vi "Common_Socket_Cmd_Sub_VI_TestMode.vi"(6 "Common Socket Error in":errorcluster, 8 "Operation Message Length":i32, 9 "Operation Message ID":i32, 11 "connection ID":refnum<k5>) -> (1 "error output":errorcluster, 3 "connection ID":refnum<k5>)   [LabVIEW 2017]
panel:
  out "Rest of the binary string":string
  out "bytes written":i32
  # "INPUT :"
  # "OUTPUT :"
  # "For Info :"
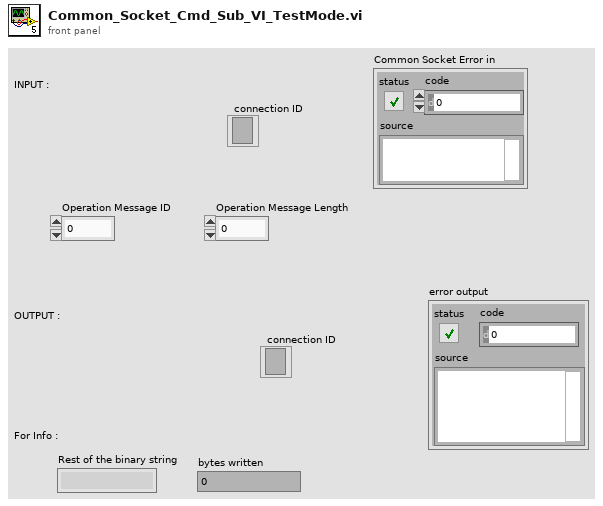
[diagram p1: front panel]
types:
  T1 = enum16{"big-endian, network order", "native, host order", "little-endian"}
  T2 = cluster{"Operation Message Length":i32, "Operation Message ID":i32}
  T3 = enum16{"Standard", "Buffered", "CRLF", "Immediate"}
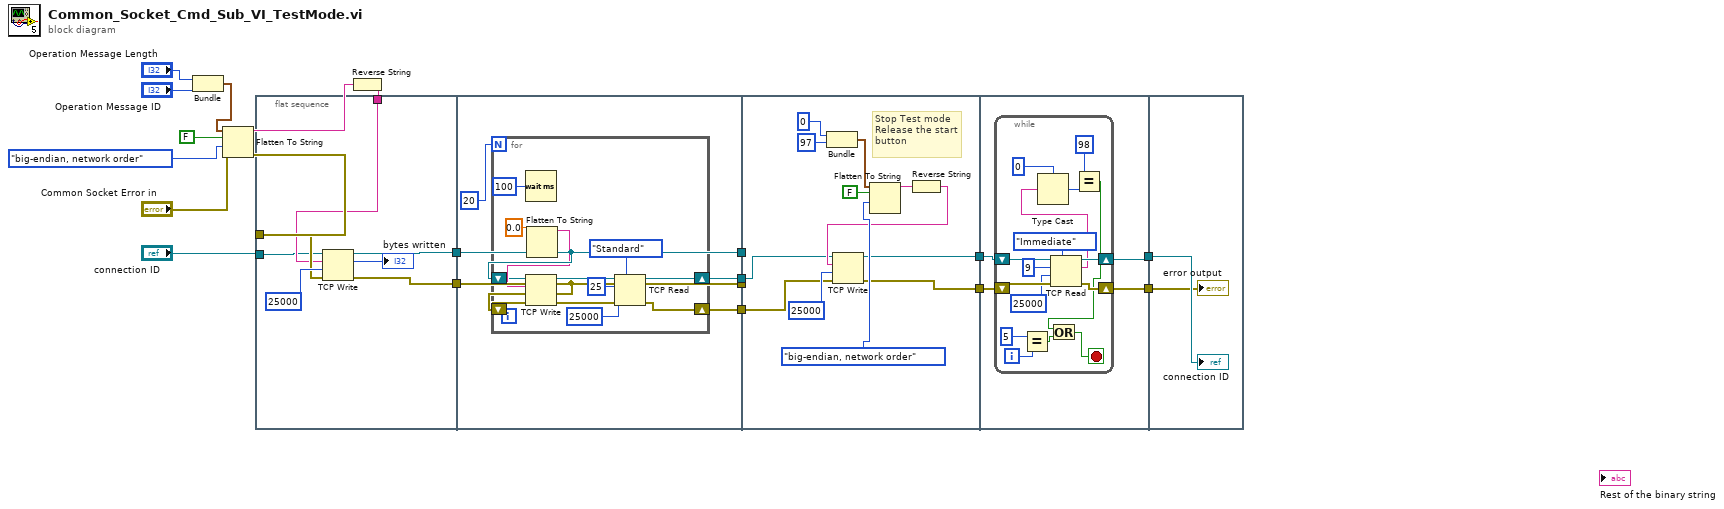
[diagram p0: block diagram]
diagram:
  n1 = Bundle("Operation Message Length"="Operation Message Length", "Operation Message ID"="Operation Message ID") -> (w13:T2)  [unwired: 1 in]
  n2 = Flatten To String(anything=w13, prepend array or string size? (T)=FALSE, byte order (0:big-endian, network order)=T1."big-endian, network order", error in (no error)="Common Socket Error in") -> (data string=w16:string, error out=w17:errorcluster)  [unwired: 1 out]
  n3 = flat-sequence {
    tunnel: [w25] -> w10
    tunnel: [w24] -> w8
    tunnel: w17 -> [w23]
    tunnel: w15 -> [w22]
    tunnel: "connection ID" -> [w21]
    tunnel: w10 -> [w32]
    tunnel: [w32] -> w9
    tunnel: w8 -> [w31]
    tunnel: [w31] -> w7
    tunnel: [w29] -> w6
    tunnel: [w28] -> w5
    tunnel: w9 -> [_]
    tunnel: w7 -> [_]
    tunnel: [w48] -> w4
    tunnel: [w47] -> w2
    tunnel: w6 -> [w46]
    tunnel: w5 -> [w45]
    tunnel: w4 -> [w60]
    tunnel: [w58] -> w3
    tunnel: w2 -> [w59]
    tunnel: [w57] -> w1
    tunnel: w3 -> [w78]
    tunnel: w1 -> [w77]
    frame #0 {
      n4 = TCP Write(connection ID=w21, data in=w22, error in (no error)=w23, 9:25000 ("timeout ms (25000)")) -> (connection ID out=w25:refnum<k5>, bytes written=→"bytes written":i32, error out=w24:errorcluster)
    }
    frame #1 {
      n5 = for {
        N: 20 -> [_]
        shift-right: [w38] -> w29
        shift-left: w32 -> [w43]
        shift-right: [w36] -> w28
        shift-left: w31 -> [w42]
        n6 = Wait (ms)(milliseconds to wait=u32 100) -> ()  [unwired: 1 out]
        n7 = Flatten To String(anything=0.0) -> (data string=w44:string)  [unwired: 3 in, 2 out]
        n8 = TCP Write(connection ID=w43, data in=w44, error in (no error)=w42) -> (connection ID out=w39:refnum<k5>, error out=w37:errorcluster)  [unwired: 1 in, 1 out]
        n9 = TCP Read(connection ID=w39, bytes to read=25, error in (no error)=w37, 7:T3."Standard" ("mode (standard)"), 9:25000 ("timeout ms (25000)")) -> (connection ID out=w38:refnum<k5>, error out=w36:errorcluster)  [unwired: 1 out]
      }
    }
    frame #2 {
      # "Stop Test mode\nRelease the start\nbutton"
      n10 = Bundle(0, 97) -> (w55:cluster{i32, i32})  [unwired: 1 in]
      n11 = Flatten To String(anything=w55, prepend array or string size? (T)=FALSE, byte order (0:big-endian, network order)=T1."big-endian, network order") -> (data string=w56:string)  [unwired: 1 in, 2 out]
      n12 = Reverse String(1:w56) -> (0:w50:string)
      n13 = TCP Write(connection ID=w46, data in=w50, error in (no error)=w45, 9:25000 ("timeout ms (25000)")) -> (connection ID out=w48:refnum<k5>, error out=w47:errorcluster)  [unwired: 1 out]
    }
    frame #3 {
      n14 = while {
        shift-right: [w74] -> w58
        shift-left: w60 -> [w76]
        shift-right: [w73] -> w57
        shift-left: w59 -> [w75]
        i -> [w69]
        stop <- w66 stop-if-true
        n15 = Equal?(x=5, y=w69) -> (x = y?=w67:bool)
        n16 = TCP Read(connection ID=w76, bytes to read=9, error in (no error)=w75, 7:T3."Immediate" ("mode (standard)"), 9:25000 ("timeout ms (25000)")) -> (connection ID out=w74:refnum<k5>, data out=w65:string, error out=w73:errorcluster)
        n17 = Type Cast(type=u8 0 ("milliseconds to wait"), x=w65) -> (*(type *) &x=w63:u8)
        n18 = Equal?(x=u32 98, y=w63) -> (x = y?=w61:bool)
        n19 = Or(x=w61, y=w67) -> (x .or. y?=w66:bool)
      }
    }
    frame #4 {
      "error output" <- w77
      "connection ID" <- w78
    }
  }
  n20 = Reverse String(1:w16) -> (0:w15:string)
